vi "Stop Measurement.vi"(8 "error in (no error)":errorcluster, 11 "Keithley Source in":refnum<class "Keithley Source.lvclass">) -> (0 "error out":errorcluster, 3 "Keithley Source out":refnum<class "Keithley Source.lvclass">)   [LabVIEW 2015, in "Keithley Source.lvclass"]
uses:
  Keithley Source.lvclass
  Instrument/Read VISA Resource.vi
  Instrument/Write VISA Resource.vi
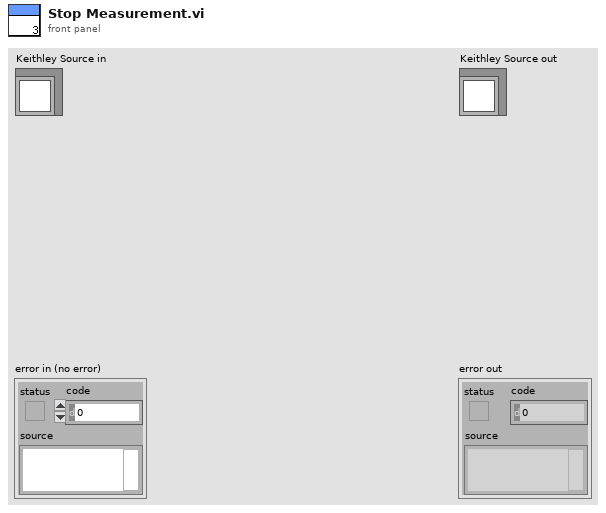
[diagram p1: front panel]
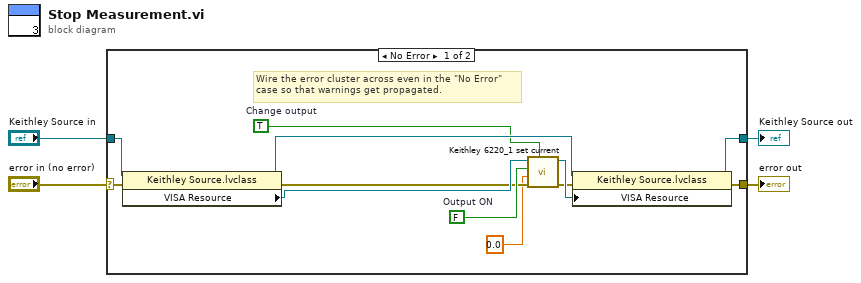
[diagram p0: block diagram]
diagram:
  n1 = case shown="No Error" "error in (no error)" {
    selector: "error in (no error)" -> [w6 w18]
    tunnel: [w9 w18] -> w3
    tunnel: [w10 w17] -> w1
    tunnel: "Keithley Source in" -> [w11 w17]
    frame No Error {
      w13 = FALSE  # Output ON
      w14 = TRUE  # Change output
      # "Wire the error cluster across even in the \"No Error\"\ncase so that warnings get propagated."
      n2 = property class="Keithley Source.lvclass"(reference=w11, error in=w6) -> (reference out=w16:refnum<class "Keithley Source.lvclass">, error out=w7:errorcluster, "VISA Resource"=w15:refnum<visa-resource-name>)
      n3 = call "Keithley 6220_1 set current.vi"("Change output"=w14, "error in (no error)"=w7, "Current (A)"=0.0, "Output ON"=w13, "VISA resource name"=w15) -> ("error out"=w8:errorcluster, "VISA resource name out"=w12:refnum<visa-resource-name>)  [unwired: 5 in]
      n4 = property class="Keithley Source.lvclass"(reference=w16, error in=w8, "VISA Resource"=w12) -> (reference out=w10:refnum<class "Keithley Source.lvclass">, error out=w9:errorcluster)
    }
    frame Error {
    }
  }
  "error out" <- w3
  "Keithley Source out" <- w1
